vi "Initialize PDF Report.vi"(0 "PDF Path":path, 5 "Unit (default = mm)":T8=enum."mm", 9 "Captions":T1={"Figure"={"Caption"="", "Separator"="", "Position"=enum."Above"}, "Table"={"Caption"="", "Separator"="", "Position"=enum."Above"}, "Font"={"Name"="", "Size"=-1.0, "Color"=0, "Style"={"Bold"=FALSE, "Italic"=FALSE, "Underline"=FALSE, "Strikeout"=FALSE}, "Type"={"Type&direction"=enum."Select", "Embedded"=FALSE, "Encoding"=""}}}, 11 "error in (no error)":errorcluster) -> (4 "PDF Report":refnum<class "PDF Report Class.lvclass">, 15 "error out (no error)":errorcluster)   [LabVIEW 2020, in "Exaprom PDF.lvlib" / "PDF Report Class.lvclass"]
doc: "Initialize the Xcontrol \"PDF Report\".\n\nVersion 1.0\nDeveloped by Jean-Marc Simard\nCopyright © 2010, Exaprom Inc.\nAll rights reserved.\nLicense: BSD\n\nWith iTextSharp 4.1.6 (http://itextsharp.sourceforge.net)\nunder Mozilla Public License Version 1.1\n(http://www.mozilla.org/MPL/MPL-1.1.html)"
uses:
  <userlib>/labview-PDF-writer-master/LV Class/PDF Report Class/PDF Report Class.lvclass
  <userlib>/labview-PDF-writer-master/Controls/Initialization Controls/Unit.ctl
  <userlib>/labview-PDF-writer-master/Controls/Initialization Controls/Captions.ctl
  <userlib>/labview-PDF-writer-master/Controls/Initialization Controls/Image or Table Caption.ctl
  <userlib>/labview-PDF-writer-master/Controls/Font Controls/Font complete cluster.ctl
  <userlib>/labview-PDF-writer-master/Controls/Font Controls/Font size.ctl
  <userlib>/labview-PDF-writer-master/Controls/Font Controls/Font color.ctl
  <userlib>/labview-PDF-writer-master/Controls/Font Controls/Type and encoding.ctl
  <userlib>/labview-PDF-writer-master/Controls/Text Controls/Unicode/Type and run direction.ctl
  <userlib>/labview-PDF-writer-master/Controls/Initialization Controls/Defaut Paragraphe and Line Spacing.ctl
  <userlib>/labview-PDF-writer-master/Controls/Text Controls/Texte alignement.ctl
  <userlib>/labview-PDF-writer-master/Controls/Text Controls/Line spacing.ctl
  <userlib>/labview-PDF-writer-master/Controls/Page Controls/Page dimensions.ctl
  <userlib>/labview-PDF-writer-master/Controls/Page Controls/Page size.ctl
  <userlib>/labview-PDF-writer-master/Controls/Page Controls/Page Orientation.ctl
  <userlib>/labview-PDF-writer-master/Controls/Header, Footer and Watermark Controls/Watermark cluster2.ctl
  <userlib>/labview-PDF-writer-master/Controls/Header, Footer and Watermark Controls/Watermark Position.ctl
  <userlib>/labview-PDF-writer-master/Controls/Header, Footer and Watermark Controls/Header footer horiz alignment.ctl
  <userlib>/labview-PDF-writer-master/LV Class/Header and Footer Class/Header and Footer Class.lvclass
  <userlib>/labview-PDF-writer-master/LV Class/Header and Footer Class/VIs/Controls/Header Footer cluster V2.ctl
  <userlib>/labview-PDF-writer-master/Controls/Header, Footer and Watermark Controls/Header or Footer.ctl
  <userlib>/labview-PDF-writer-master/Controls/Header, Footer and Watermark Controls/Header Footer Type.ctl
  <userlib>/labview-PDF-writer-master/Controls/Table Controls/Cell Vertical alignment.ctl
  <userlib>/labview-PDF-writer-master/Controls/Header, Footer and Watermark Controls/Page number.ctl
  <userlib>/labview-PDF-writer-master/Controls/Font Controls/Font complete cluster horizontal.ctl
  <userlib>/labview-PDF-writer-master/Controls/Header, Footer and Watermark Controls/Header Footer Line.ctl
  <userlib>/labview-PDF-writer-master/LV Class/PDF Report Class/PDF Report Class.lvclass/PDF Report Class.ctl
  C:/Program Files (x86)/National Instruments/LabVIEW 2020/user.lib/labview-PDF-writer-master/DLL/itextsharp.dll
  DLL/itextsharp.dll
  <userlib>/labview-PDF-writer-master/Exaprom PDF.lvlib
  <userlib>/labview-PDF-writer-master/LV Class/Fonts Class/Font Class.lvclass
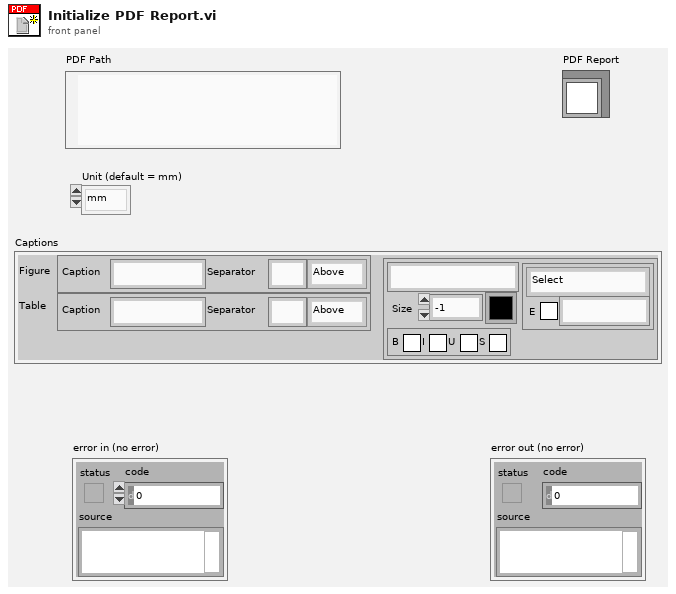
[diagram p1: front panel]
types:
  T1 = typedef "Exaprom PDF.lvlib/Captions.ctl" = cluster{"Figure":T2, "Table":T2, "Font":T3}
  T2 = typedef "Exaprom PDF.lvlib/Image or Table Caption.ctl" = cluster{"Caption":string, "Separator":string, "Position":enum16{"Above", "Below"}}
  T3 = typedef "Exaprom PDF.lvlib/Font complete cluster.ctl" = cluster{"Name":string, "Size":T4, "Color":T5, "Style":cluster{"Bold":bool, "Italic":bool, "Underline":bool, "Strikeout":bool}, "Type":T6}
  T4 = typedef "Exaprom PDF.lvlib/Font size.ctl" = sgl
  T5 = typedef "Exaprom PDF.lvlib/Font color.ctl" = u32
  T6 = typedef "Exaprom PDF.lvlib/Type and encoding.ctl" = cluster{"Type&direction":T7, "Embedded":bool, "Encoding":string}
  T7 = typedef "Exaprom PDF.lvlib/Type and run direction.ctl" = enum16{"Select", "ASCII", "UTF-16", "UTF-16 (default)", "UTF-16 (LTR)", "UTF-16 (RTL)"}
  T8 = typedef "Exaprom PDF.lvlib/Unit.ctl" = enum16{"inch", "mm"}
  T9 = typedef "Exaprom PDF.lvlib/Header and Footer Class.lvclass/Header Footer cluster V2.ctl" = cluster{"Header or Footer":T10, "Start page":i32, "Start with #":i32, "Type":T11, "Alignment":T12, "Vertical Alignement":T13, "Line spacing":T14, "Image (%)":sgl, "Page #":T15, "Text":string, "Path":string, "Font":T16, "Font refnum":refnum<k24>, "Line":cluster{"Line":T17, "Thickness (points)":sgl, "Colour":T5}, "Vert margin":dbl, "Hyperlink":string}
  T10 = typedef "Exaprom PDF.lvlib/Header or Footer.ctl" = enum16{"Header", "Footer"}
  T11 = typedef "Exaprom PDF.lvlib/Header Footer Type.ctl" = enum16{"Select", "Text", "Text + hyperlink", "Page number", "Image", "Image + hyperlink"}
  T12 = typedef "Exaprom PDF.lvlib/Header footer horiz alignment.ctl" = enum16{"Left", "Center", "Right"}
  T13 = typedef "Exaprom PDF.lvlib/Cell Vertical alignment.ctl" = enum16{"TOP", "MIDDLE", "BOTTOM"}
  T14 = typedef "Exaprom PDF.lvlib/Line spacing.ctl" = enum16{"Select", "1.0", "1.5", "2.0"}
  T15 = typedef "Exaprom PDF.lvlib/Page number.ctl" = cluster{"Text 1":string, "Text 2":string, "Text 3":string}
  T16 = typedef "Exaprom PDF.lvlib/Font complete cluster horizontal.ctl" = cluster{"Name":string, "Size":T4, "Color":T5, "Style":cluster{"Bold":bool, "Italic":bool, "Underline":bool, "Strikeout":bool}, "Type":T6}
  T17 = typedef "Exaprom PDF.lvlib/Header Footer Line.ctl" = enum16{"No line", "Horizontal line"}
  T18 = typedef "Exaprom PDF.lvlib/Watermark cluster2.ctl" = cluster{"Show? (F)":bool, "Type":enum16{"Image", "Text"}, "Opacity (%)":sgl, "Rotate(°)":sgl, "Position":cluster{"Position":T19, "X":sgl, "Y":sgl}, "Image path":path, "Scaled(%)":sgl, "Image refnum":refnum<k24>, "Text":string, "Font":cluster{"Name":string, "Size":T4, "Color":T5}, "Font refnum":refnum<k24>, "Alignment":T12, "Automatic":bool}
  T19 = typedef "Exaprom PDF.lvlib/Watermark Position.ctl" = enum16{"Absolute", "Center (page)", "Center (text section)"}
  T20 = typedef "Exaprom PDF.lvlib/Page dimensions.ctl" = cluster{"Start at page":i32, "Page Size":T21, "Orientation":T22, "widht":sgl, "height":sgl, "Margin left":sgl, "Margin right":sgl, "Margin top":sgl, "Margin bottom":sgl, "X0":sgl, "X1":sgl, "Y0":sgl, "Y1":sgl}
  T21 = typedef "Exaprom PDF.lvlib/Page size.ctl" = i32
  T22 = typedef "Exaprom PDF.lvlib/Page Orientation.ctl" = enum16{"Portrait", "Landscape"}
  T23 = typedef "Exaprom PDF.lvlib/Defaut Paragraphe and Line Spacing.ctl" = cluster{" Aligment":T24, "Line spacing":T14}
  T24 = typedef "Exaprom PDF.lvlib/Texte alignement.ctl" = enum16{"Select", "CENTER", "JUSTIFY", "LEFT", "RIGHT"}
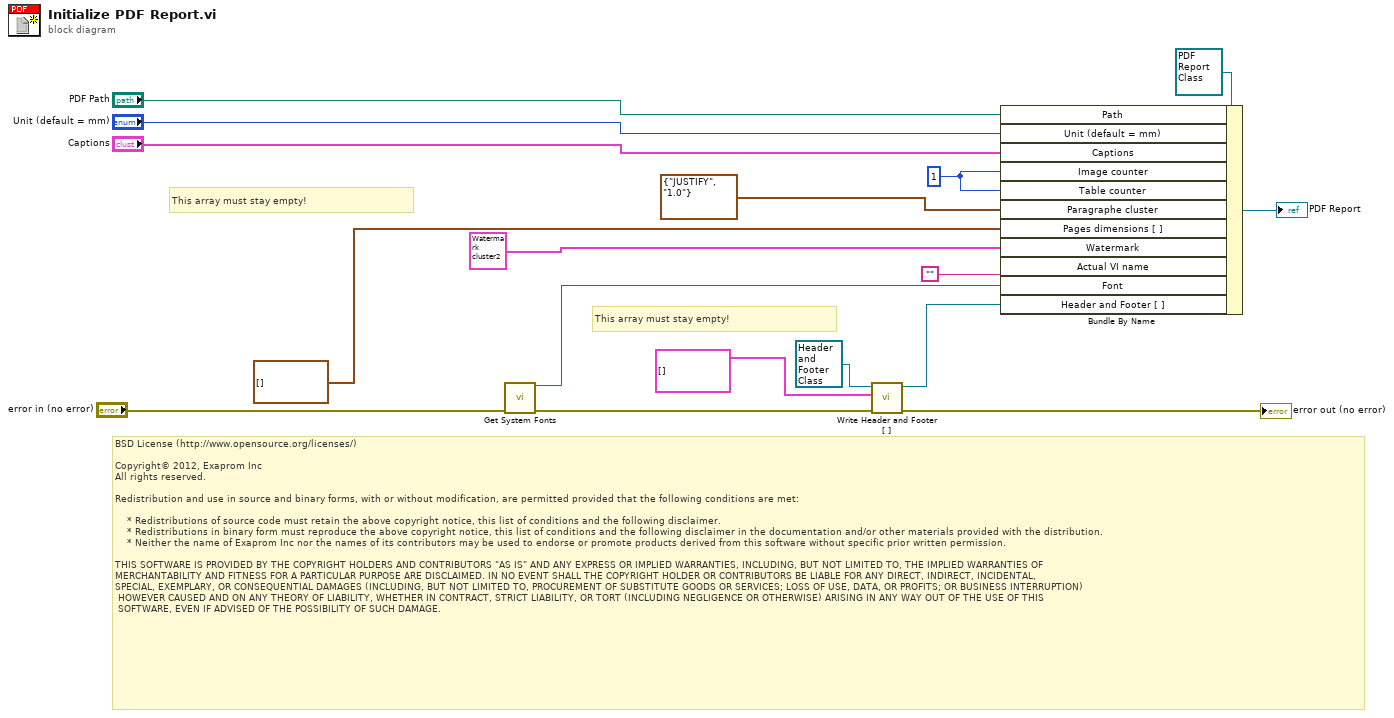
[diagram p0: block diagram]
diagram:
  w7 = u16 1 ("Captions.Image counter")
  # "This array must stay empty!"
  # "This array must stay empty!"
  # "BSD License (http://www.opensource.org/licenses/)\n\nCopyright© 2012, Exaprom Inc\nAll rights reserved.\n\nRedistribution and use in source and binary forms, with or without modification, are permitted provided that the following conditions are met:\n\n    * Redistributions of source code must retain the above copyright notice, this list of conditions and the following disclaimer.\n    * Redistributions in binary form must reproduce the above copyright notice, this list of conditions and the following disclaimer in the documentation and/or other materials provided with the distribution.\n    * Neither the name of Exaprom Inc nor the names of its contributors may be used to endorse or promote products derived from this software without specific prior written permission.\n\nTHIS SOFTWARE IS PROVIDED BY THE COPYRIGHT HOLDERS AND CONTRIBUTORS \"AS IS\" AND ANY EXPRESS OR IMPLIED WARRANTIES, INCLUDING, BUT NOT LIMITED TO, THE IMPLIED WARRANTIES OF \nMERCHANTABILITY AND FITNESS FOR A PARTICULAR PURPOSE ARE DISCLAIMED. IN NO EVENT SHALL THE COPYRIGHT HOLDER OR CONTRIBUTORS BE LIABLE FOR ANY DIRECT, INDIRECT, INCIDENTAL,\nSPECIAL, EXEMPLARY, OR CONSEQUENTIAL DAMAGES (INCLUDING, BUT NOT LIMITED TO, PROCUREMENT OF SUBSTITUTE GOODS OR SERVICES; LOSS OF USE, DATA, OR PROFITS; OR BUSINESS INTERRUPTION)\n HOWEVER CAUSED AND ON ANY THEORY OF LIABILITY, WHETHER IN CONTRACT, STRICT LIABILITY, OR TORT (INCLUDING NEGLIGENCE OR OTHERWISE) ARISING IN ANY WAY OUT OF THE USE OF THIS\n SOFTWARE, EVEN IF ADVISED OF THE POSSIBILITY OF SUCH DAMAGE."
  n1 = call <userlib>:"Get System Fonts.vi"("error in (no error)"="error in (no error)") -> ("Font OUT"=w5:refnum<class "Font Class.lvclass">, "error out"=w4:errorcluster)  [unwired: 13 in]
  n2 = call-dynamic "Write Header and Footer [ ].vi"("error in (no error)"=w4, "Header and Footer [ ]"=T9[] [], "Header and Footer Class in"=refnum<class "Header and Footer Class.lvclass"> refnum) -> ("error out"=→"error out (no error)":errorcluster, "Header and Footer Class out"=w2:refnum<class "Header and Footer Class.lvclass">)  [unwired: 7 in]
  n3 = Bundle By Name(cluster=refnum<class "PDF Report Class.lvclass"> refnum ("PDF Report Class.lvclass"), "Path"="PDF Path", "Unit (default = mm)"="Unit (default = mm)", "Captions"="Captions", "Image counter"=w7, "Table counter"=w7, "Paragraphe cluster"=T23 {" Aligment"=enum."JUSTIFY", "Line spacing"=enum."1.0"} ("Value"), "Pages dimensions [ ]"=T20[] [] ("Page dimensions [ ]"), "Watermark"=T18 {"Show? (F)"=FALSE, "Type"=enum."Text", "Opacity (%)"=10.0, "Rotate(°)"=0.0, "Position"={"Position"=enum."Center (text section)", "X"=0.0, "Y"=0.0}, "Image path"=path "", "Scaled(%)"=100.0, "Image refnum"=refnum, "Text"="CONFIDENTIAL", "Font"={"Name"="", "Size"=-1.0, "Color"=0}, "Font refnum"=refnum, "Alignment"=enum."Left", "Automatic"=FALSE}, "Actual VI name"="", "Font"=w5, "Header and Footer [ ]"=w2) -> (→"PDF Report":refnum<class "PDF Report Class.lvclass">)
